vi "time_step_attempt_with_pressure_with_safety_off.vi"() -> ()   [LabVIEW 2017]
uses:
  <vilib>/Waveform/WDTFileIO.llb/Export Waveforms To Spreadsheet File (1D).vi
panel:
  in  "Displacement Scale (mm/V)":dbl
  out "Disp":dynamicdata(graph)
  out "Measured pressure":dynamicdata(graph)
  in  "Pressure Target psi":dbl min=0.0 max=750.0 step=10.0
  in  "Time to hold at start value":dbl
  out "Current value":i32
  in  "Number of cycles":i32
  out "Number of steps":i32
  out "Number of cycles":i32
  in  "End value":i32
  in  "Start value":i32
  in  "Step value":i32
  in  "Seconds between steps":dbl
  in  "stop":bool
  out "current ref time":timestamp
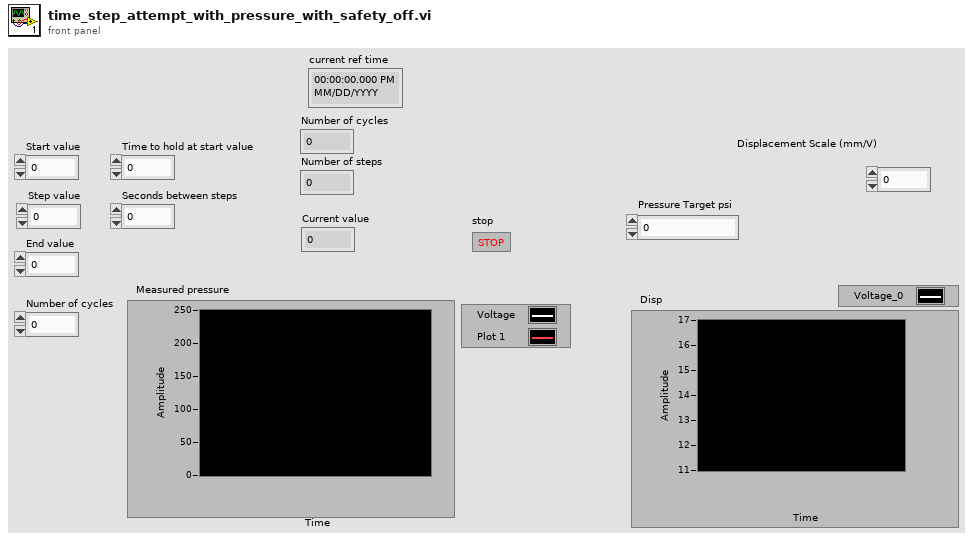
[diagram p1: front panel]
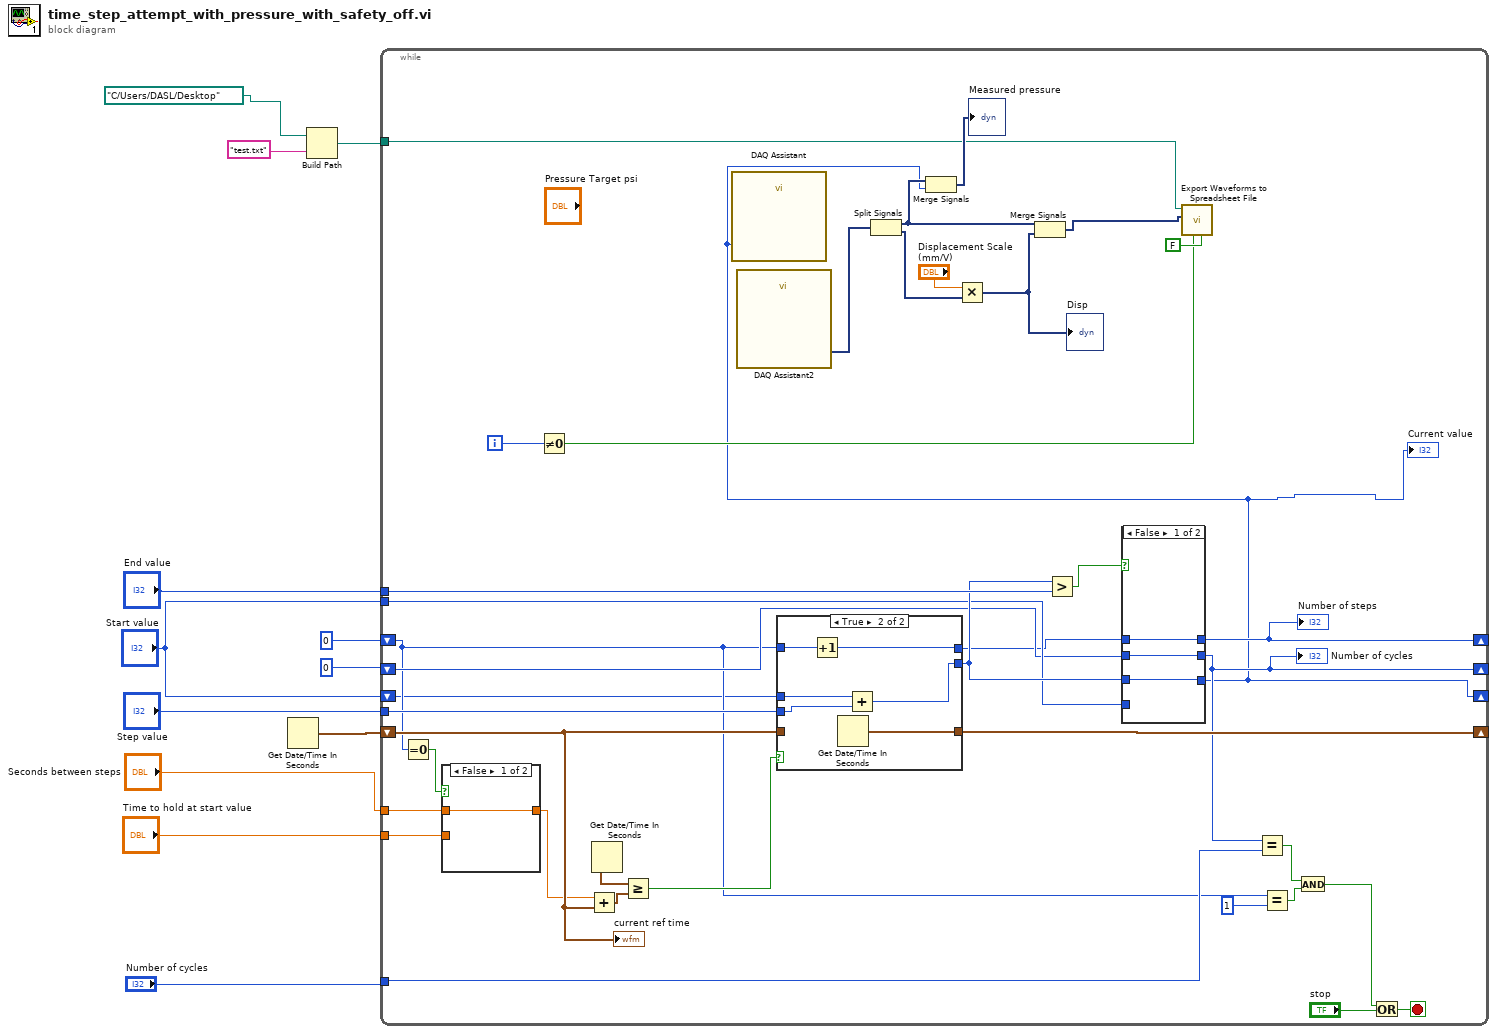
[diagram p0: block diagram]
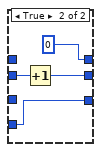
[diagram p3: hidden frame]
diagram:
  n1 = Get Date/Time In Seconds() -> (seconds since 1Jan1904=w11:timestamp)
  n2 = Build Path(base path=path "C:/Users/DASL/Desktop", name or relative path="test.txt") -> (appended path=w1:path)
  n3 = while {
    shift-right: [w13] -> _
    shift-left: "Start value" -> [w27]
    tunnel: "Step value" -> [w48]
    shift-right: [w47] -> _
    shift-left: w11 -> [w46]
    tunnel: "Seconds between steps" -> [w32]
    shift-right: [w36] -> _
    shift-left: 0 -> [w30]
    tunnel: "End value" -> [w45]
    tunnel: "Start value" -> [w42]
    shift-right: [w40] -> _
    shift-left: 0 -> [w41]
    tunnel: "Number of cycles" -> [w39]
    tunnel: "Time to hold at start value" -> [w33]
    tunnel: w1 -> [w16]
    i -> [w15]
    stop <- w25 stop-if-true
    n4 = Equal To 0?(x=w30) -> (x = 0?=w35:bool)
    n5 = case shown="False" w35 {
      tunnel: [w52 w53] -> w34
      tunnel: w33 -> [_ w53]
      tunnel: w32 -> [w52 _]
      frame False {
      }
      frame True {
      }
    }
    n6 = Not Equal To 0?(x=w15) -> (x != 0?=w14:bool)
    n7 = Add(x=w34, y=w46) -> (x+y=w51:timestamp)
    n8 = Get Date/Time In Seconds() -> (seconds since 1Jan1904=w50:timestamp)
    n9 = Greater Or Equal?(x=w50, y=w51) -> (x >= y?=w49:bool)
    n10 = call "DAQ Assistant2"() -> ("data"=w22:dynamicdata)  [unwired: 17 in, 2 out]
    n11 = case shown="True" w49 {
      tunnel: w27 -> [w63 w69]
      tunnel: [w63 w67] -> w43
      tunnel: w48 -> [_ w68]
      tunnel: [w61 w66] -> w47
      tunnel: [w62 w65] -> w37
      tunnel: w30 -> [w62 w64]
      tunnel: w46 -> [w61 _]
      frame False {
      }
      frame True {
        n12 = Increment(x=w64) -> (x+1=w65:i32)
        n13 = Get Date/Time In Seconds() -> (seconds since 1Jan1904=w66:timestamp)
        n14 = Add(x=w69, y=w68) -> (x+y=w67:i32)
      }
    }
    n15 = Split Signals(w22) -> (w21:dynamicdata, w20:dynamicdata)  [unwired: 2 in]
    n16 = Multiply(x="Displacement Scale (mm/V)", y=w20) -> (x*y=w23:dynamicdata)
    "Disp" <- w23
    n17 = Merge Signals(w21, w23) -> (w19:dynamicdata)
    n18 = Greater?(x=w43, y=w45) -> (0:w44:bool)
    n19 = case shown="False" w44 {
      tunnel: w43 -> [w56 _]
      tunnel: [w56 w60] -> w13
      tunnel: w42 -> [_ w60]
      tunnel: [w55 w59] -> w40
      tunnel: w41 -> [w55 w58]
      tunnel: w37 -> [w54 _]
      tunnel: [w54 0] -> w36
      frame False {
      }
      frame True {
        n20 = Increment(x=w58) -> (x+1=w59:i32)
      }
    }
    "Number of cycles" <- w40
    "Number of steps" <- w36
    "Current value" <- w13
    n21 = call "DAQ Assistant"("data"=w13) -> ()  [unwired: 17 in, 2 out]
    n22 = Merge Signals(w21, w13) -> (→"Measured pressure":dynamicdata)
    n23 = call-poly <vilib>:"Export Waveforms to Spreadsheet File.vi"("header? (write header:T)"=FALSE, "append to file? (new file:F)"=w14, "waveforms"=w19, "file path (dialog if empty)"=w16) -> ()  [unwired: 6 in, 2 out]
    n24 = Equal?(x=w40, y=w39) -> (x = y?=w31:bool)
    n25 = Equal?(x=w30, y=1) -> (x = y?=w28:bool)
    n26 = And(x=w31, y=w28) -> (x .and. y?=w26:bool)
    n27 = Or(x=w26, y="stop") -> (x .or. y?=w25:bool)
    "current ref time" <- w46
  }
